vi "MT Demodulate MSK.vi"(0 "input complex waveform":T1={"t0"=0.0, "dt"=1.0, "Y"=[]} {"Y" format="%.3f"; "dt" format="%^.2e"; "t0" format="%.4f"}, 5 "MSK system parameters":T4={"differential encoding enable"=enum."enable", "samples per symbol (16)"=16}, 7 "matched filter coefficients":dbl[](array[numeric]) format="%.2f", 9 "synchronization parameters":T3 {"sync sequence" format="%.2f"}, 11 "error in (no error)":errorcluster, 12 "pulse shaping filter coefficients":dbl[](array[numeric]) format="%.2f", 13 "reset? (T)":bool=TRUE) -> (3 "detected complex waveform":cluster{"t0":dbl, "dt":dbl, "Y":cdb[]} {"Y" format="%.3f"; "dt" format="%^.2e"; "t0" format="%.4f"}, 4 "recovered complex waveform":T1 {"Y" format="%.3f"; "dt" format="%^.2e"; "t0" format="%.4f"}, 6 "output bit stream":i8[](array[numeric]), 8 "measurements":T2 {"frequency drift (Hz)" format="%.2f"; "frequency offset (Hz)" format="%.2f"}, 10 "sync found index (symbols)":dbl format="%.4f", 15 "error out":errorcluster)   [LabVIEW 2020, in "niDMT.lvlib"]
doc: "Demodulates an minimum shift keying (MSK)-modulated complex baseband waveform and returns the time-aligned oversampled complex waveform, the ideal oversampled waveform, the demodulated bit stream, and the results of offset and drift measurements. This VI attempts to remove carrier and phase offset by locking to the carrier signal."
uses:
  <vilib>/addons/Modulation/niDMT.lvlib
  <vilib>/addons/Modulation/Analog/controls/Complex Data Waveform.ctl
  <vilib>/addons/Modulation/Analog/MT Resample (Complex Cluster).vi
  <vilib>/addons/Modulation/Analog/support/Validators/mod_Fractional Resample Validate.vi
  <vilib>/addons/Modulation/Analog/support/Validators/mod_Check Flush State.vi
  <vilib>/addons/Modulation/Analog/support/mod_FractionalResampler.vi
  <vilib>/addons/Modulation/Analog/support/mod_Integer Rate Interpolation.vi
  <vilib>/addons/Modulation/Analog/support/Validators/mod_Validate Complex Waveform.vi
  <vilib>/addons/Modulation/Analog/support/mod_PerformResampling.vi
  <vilib>/addons/Modulation/Analog/support/Validators/mod_WFErrorHandler.vi
  <vilib>/addons/Modulation/Digital/Support/Common/mod_Truncate FIR Filter (real).vi
  <vilib>/Utility/error.llb/Error Cluster From Error Code.vi
  <vilib>/addons/Modulation/Analog/support/mod_Resampling Factors.vi
  <vilib>/addons/Modulation/Analog/support/mod_ResamplingFilter.vi
  <vilib>/addons/Modulation/Analog/support/mod_Generate Integer Interpolation Filter.vi
  <vilib>/addons/Modulation/niAMT.lvlib
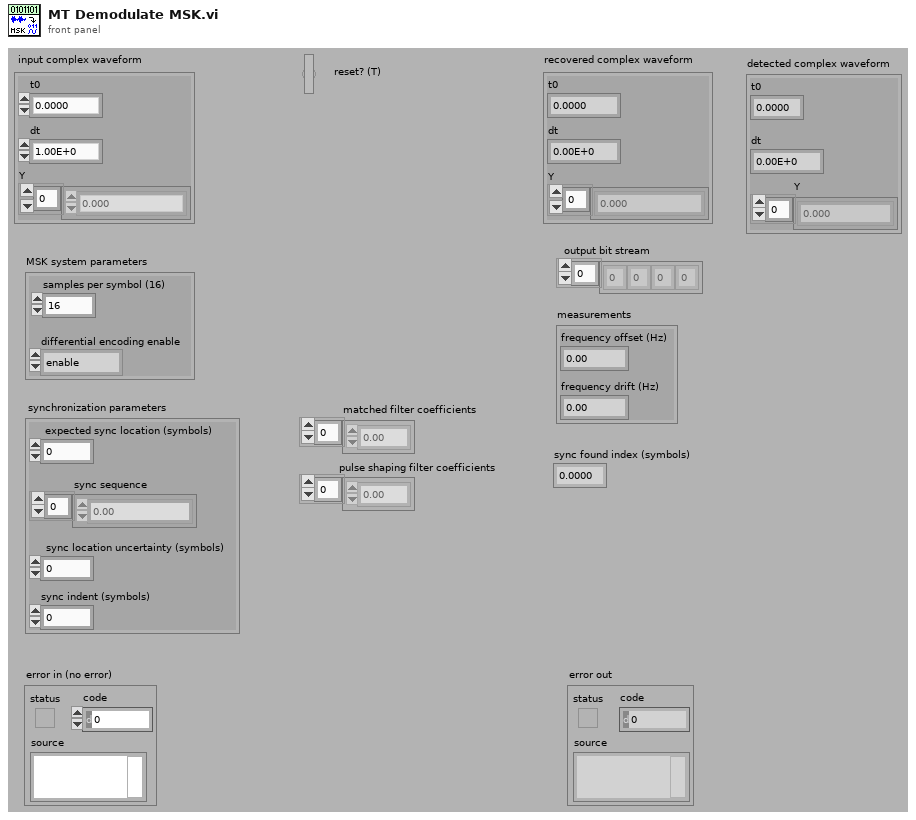
[diagram p1: front panel]
types:
  T1 = typedef "niAMT.lvlib/Complex Data Waveform.ctl" = cluster{"t0":dbl, "dt":dbl, "Y":cdb[]}
  T2 = cluster{"frequency offset (Hz)":dbl, "frequency drift (Hz)":dbl}
  T3 = cluster{"expected sync location (symbols)":i32, "sync sequence":cdb[], "sync location uncertainty (symbols)":i32, "sync indent (symbols)":i32}
  T4 = cluster{"differential encoding enable":enum16{"disable", "enable"}, "samples per symbol (16)":i32}
  T5 = enum16{"FSK", "PSK", "QAM", "MSK", "PAM", "ASK", "CPM"}
  T6 = cluster{"Frequency Estimate, Hz":dbl, "Frequency Drift, Hz":dbl}
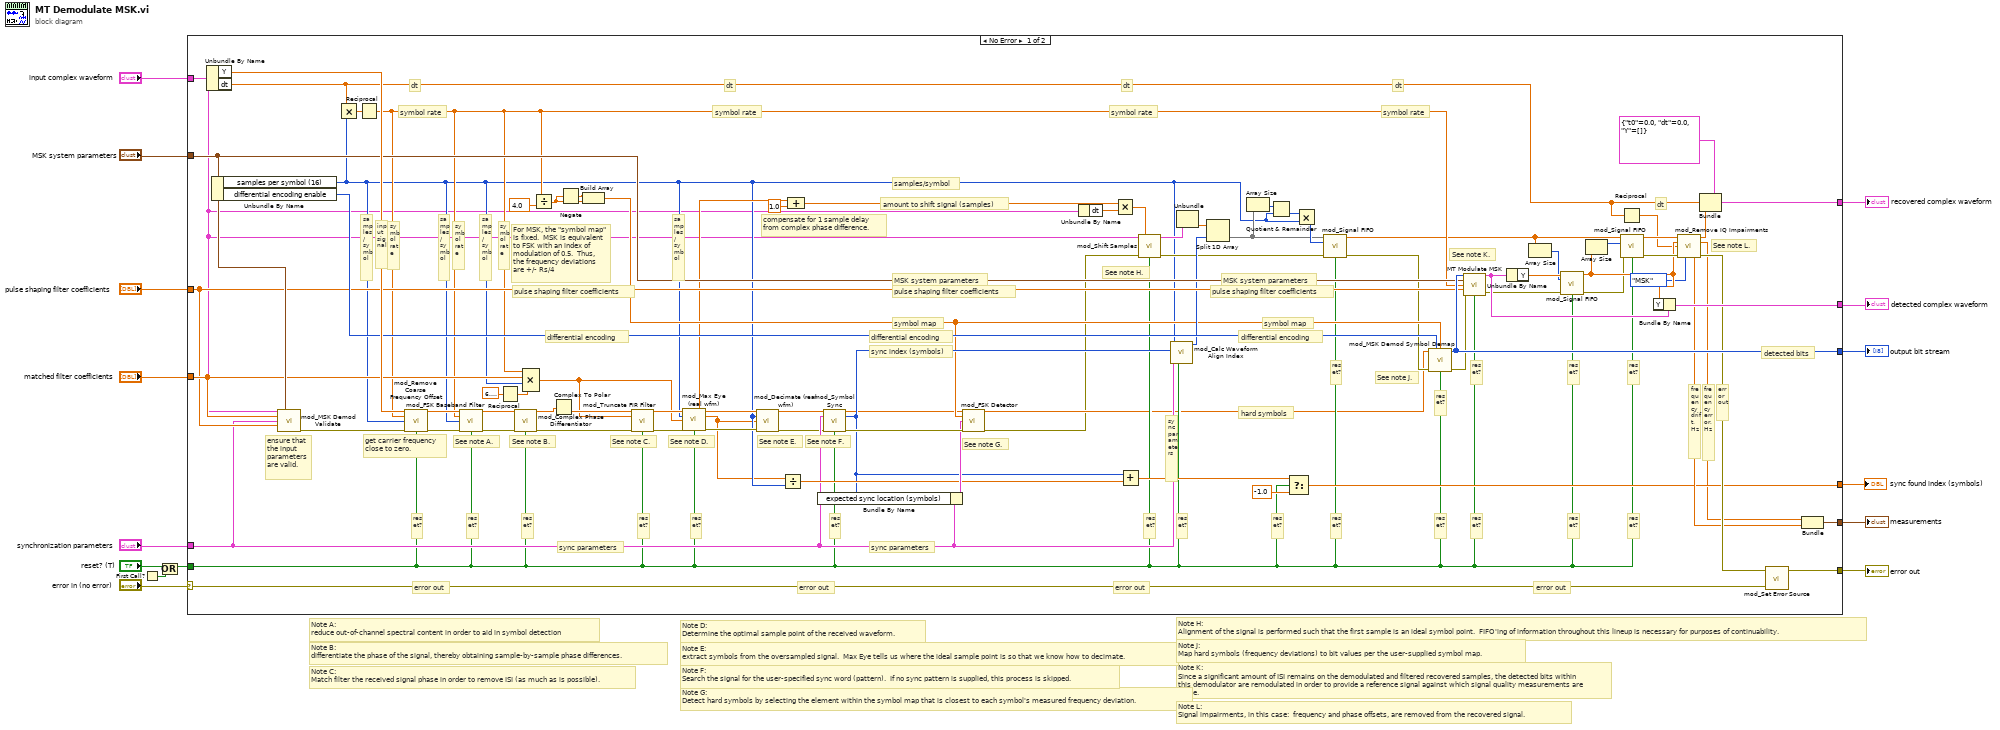
[diagram p0: block diagram]
diagram:
  # "Note A:\nreduce out-of-channel spectral content in order to aid in symbol detection"
  # "Note B:\ndifferentiate the phase of the signal, thereby obtaining sample-by-sample phase differences."
  # "Note C:\nMatch filter the received signal phase in order to remove ISI (as much as is possible)."
  # "Note D:\nDetermine the optimal sample point of the received waveform."
  # "Note E:\nextract symbols from the oversampled signal.  Max Eye tells us where the ideal sample point is so that we know how to decimate."
  # "Note F:\nSearch the signal for the user-specified sync word (pattern).  If no sync pattern is supplied, this process is skipped."
  # "Note G:\nDetect hard symbols by selecting the element within the symbol map that is closest to each symbol's measured frequency deviation."
  # "Note H:\nAlignment of the signal is performed such that the first sample is an ideal symbol point.  FIFO'ing of information throughout this lineup is necessary for purposes of continuability."
  # "Note J:\nMap hard symbols (frequency deviations) to bit values per the user-supplied symbol map."
  # "Note K:\nSince a significant amount of ISI remains on the demodulated and filtered recovered samples, the detected bits within this demodulator are remodulated in order to provide a reference signal against which signal quality measurements are made."
  # "Note L:\nSignal impairments, in this case:  frequency and phase offsets, are removed from the recovered signal."
  n1 = First Call?() -> (First Call?: T/F=w3:bool)
  n2 = Or(x="reset? (T)", y=w3) -> (x .or. y?=w1:bool)
  n3 = case shown="No Error" "error in (no error)" {
    selector: "error in (no error)" -> [w80 w98]
    tunnel: [w81 w98] -> w7
    tunnel: "synchronization parameters" -> [w63 _]
    tunnel: "matched filter coefficients" -> [w67 _]
    tunnel: "MSK system parameters" -> [w68 _]
    tunnel: "pulse shaping filter coefficients" -> [w66 _]
    tunnel: [w37 _] -> w8
    tunnel: "input complex waveform" -> [w17 _]
    tunnel: [w91 _] -> w9
    tunnel: [w88 _] -> w6
    tunnel: w1 -> [w31 _]
    tunnel: [w76 _] -> w5
    tunnel: [w72 _] -> w4
    frame No Error {
      # "sync parameters"
      # "sync parameters"
      # "sync parameters"
      # "error out"
      # "error out"
      # "error out"
      # "error out"
      # "error out"
      # "frequency error, Hz"
      # "frequency drift, Hz"
      # "samples/symbol"
      # "samples/symbol"
      # "reset?"
      # "reset?"
      # "reset?"
      # "reset?"
      # "reset?"
      # "reset?"
      # "reset?"
      # "reset?"
      # "reset?"
      # "reset?"
      # "reset?"
      # "reset?"
      # "reset?"
      # "reset?"
      # "reset?"
      # "reset?"
      # "reset?"
      # "reset?"
      # "reset?"
      # "detected bits"
      # "hard symbols"
      # "MSK system parameters"
      # "pulse shaping filter coefficients"
      # "symbol map"
      # "differential encoding"
      # "pulse shaping filter coefficients"
      # "differential encoding"
      # "input signal"
      # "symbol rate"
      # "symbol rate"
      # "samples/symbol"
      # "samples/symbol"
      # "symbol rate"
      # "sync index (symbols)"
      # "amount to shift signal (samples)"
      # "samples/symbol"
      # "differential encoding"
      # "dt"
      # "symbol rate"
      # "dt"
      # "dt"
      # "symbol rate"
      # "MSK system parameters"
      # "pulse shaping filter coefficients"
      # "symbol map"
      # "symbol rate"
      # "dt"
      # "dt"
      # "For MSK, the \"symbol map\" is fixed.  MSK is equivalent to FSK with an index of modulation of 0.5.  Thus, the frequency deviations are +/- Rs/4"
      # "compensate for 1 sample delay\nfrom complex phase difference."
      # "See note A."
      # "See note B."
      # "ensure that\nthe input\nparameters\nare valid."
      # "get carrier frequency\nclose to zero."
      # "See note D."
      # "See note E."
      # "See note C."
      # "See note F."
      # "See note G."
      # "See note H."
      # "See note J."
      # "See note K."
      # "See note L."
      # "symbol rate"
      n4 = Unbundle By Name(w17) -> ("Y"=w87:cdb[], "dt"=w24:dbl)
      n5 = Unbundle By Name(w68) -> ("samples per symbol (16)"=w29:i32, "differential encoding enable"=w71:enum16{"disable", "enable"})
      n6 = call <vilib>:"mod_MSK Demod Validate.vi"("Input Complex Waveform"=w17, "MSK System Parameters"=w68, "Matched Filter Coefficients"=w67, "Synchronization Parameters"=w63, "Pulse Shaping Filter Coefficients"=w66) -> ("error out"=w69:errorcluster)  [unwired: 10 out]
      n7 = Multiply(x=w24, y=w29) -> (x*y=w89:dbl)
      n8 = Reciprocal(x=w89) -> (1/x=w30:dbl)
      n9 = call <vilib>:"mod_Remove Coarse Frequency Offset.vi"("Signal In"=w87, "Symbol Rate, Hz"=w30, "Samples Per Symbol (16)"=w29, "error in (no error)"=w69, "Reset? (T)"=w31) -> ("Signal Out"=w33:cdb[], "error out"=w35:errorcluster)  [unwired: 9 out]
      n10 = call <vilib>:"mod_FSK Baseband Filter.vi"("Signal In"=w33, "Symbol Rate, Hz"=w30, "Samples Per Symbol (16)"=w29, "error in (no error)"=w35, "Reset? (T)"=w31) -> ("Signal Out"=w32:cdb[], "error out"=w34:errorcluster)  [unwired: 9 in]
      n11 = Reciprocal(x=6.283185307179586) -> (1/x=w86:dbl)
      n12 = call <vilib>:"mod_Complex Phase Differentiator.vi"("Signal In"=w32, "error in (no error)"=w34, "Reset? (T)"=w31) -> ("Signal Out"=w54:cdb[], "error out"=w96:errorcluster)  [unwired: 11 in]
      n13 = Compound Arithmetic op=MULTIPLY(w30, w67, w29, w86) -> (w41:dbl[])
      n14 = Divide(x=w30, y=4.0) -> (x/y=w74:dbl)
      n15 = Complex To Polar(r * e^(i*theta)=w54) -> (theta=w90:dbl[])  [unwired: 1 out]
      n16 = Negate(x=w74) -> (-x=w73:dbl)
      n17 = Build Array(w73, w74) -> (w43:dbl[])
      n18 = call-poly <vilib>:"mod_Truncate FIR Filter.vi"("Signal In"=w90, "Filter Coefficients"=w41, "error in (no error)"=w96, "Reset? (T)"=w31) -> ("Signal Out"=w92:dbl[], "error out"=w95:errorcluster)  [unwired: 8 in, 2 out]
      n19 = call <vilib>:"mod_Max Eye (real wfm).vi"("Signal In"=w92, "Samples Per Symbol (16)"=w29, "Filter Coefficients"=w41, "error in (no error)"=w95, "Reset? (T)"=w31) -> ("Waveform Alignment Offset"=w42:dbl, "Signal Out"=w48:dbl[], "Optimal Offset (samples)"=w19:dbl, "error out"=w94:errorcluster)  [unwired: 6 in, 1 out]
      n20 = call <vilib>:"mod_Decimate (real wfm).vi"("Signal In"=w48, "Samples Per Symbol (16)"=w29, "Offset"=w19, "error in (no error)"=w94) -> ("Signal Out"=w44:dbl[], "error out"=w28:errorcluster)  [unwired: 10 in]
      n21 = Divide(x=w19, y=w29) -> (x/y=w65:dbl)
      n22 = Compound Arithmetic op=ADD(w42, 1.0 ("value")) -> (w40:dbl)
      n23 = call <vilib>:"mod_Symbol Sync.vi"("Signal In"=w44, "Synchronization Parameters"=w63, "error in (no error)"=w28, "Reset? (T)"=w31) -> ("Signal Out"=w36:cdb[], "Sync Location (symbols)"=w61:i32, "error out"=w97:errorcluster)  [unwired: 9 out]
      n24 = Bundle By Name(cluster=w63, "expected sync location (symbols)"=w61) -> (w83:T3)
      n25 = call <vilib>:"mod_FSK Detector.vi"("Symbols"=w36, "Symbol Map"=w43, "Synchronization Parameters"=w83, "error in (no error)"=w97) -> ("Detected Symbols"=w22:dbl[], "error out"=w18:errorcluster)  [unwired: 1 in, 9 out]
      n26 = Unbundle By Name(w17) -> ("dt"=w16:dbl)
      n27 = Multiply(x=w40, y=w16) -> (x*y=w79:dbl)
      n28 = Add(x=w61, y=w65) -> (x+y=w39:dbl)
      n29 = call <vilib>:"mod_Shift Samples.vi"("Input Complex Waveform"=w17, "Initial Sample Offset, sec"=w79, "error in (no error)"=w18, "Reset? (T)"=w31) -> ("Output Complex Waveform"=w84:T1, "error out"=w56:errorcluster)  [unwired: 10 in]
      n30 = call <vilib>:"mod_Calc Waveform Align Index.vi"("Reset? (T)"=w31, "Synchronization Parameters"=w63, "Sync Location, symbols"=w61, "Samples Per Symbol (16)"=w29) -> ("align index, samples"=w62:i32)  [unwired: 7 out]
      n31 = Unbundle(w84) -> ("Y"=w85:cdb[])  [unwired: 2 out]
      n32 = Split 1D Array(array=w85, index=w62) -> (second subarray=w57:cdb[])  [unwired: 1 out]
      n33 = Array Size(array=w57) -> (size(s)=w60:i32)
      n34 = Quotient & Remainder(x=w60, y=w29) -> (floor(x/y)=w59:i32)  [unwired: 1 out]
      n35 = Select(t=w39, s=w31, f=-1.0) -> (s? t:f=w37:dbl)
      n36 = Multiply(x=w59, y=w29) -> (x*y=w58:i32)
      n37 = call <vilib>:"mod_Signal FIFO.vi"("Signal In"=w57, "Output Length"=w58, "error in (no error)"=w56, "Reset? (T)"=w31) -> ("Signal Out"=w26:cdb[], "error out"=w27:errorcluster)  [unwired: 10 out]
      n38 = call <vilib>:"mod_MSK Demod Symbol Demap.vi"("Symbols In"=w22, "Differential Encoding Enable"=w71, "Symbol Map"=w43, "error in (no error)"=w27, "Reset? (T)"=w31) -> ("Bits Out"=w91:i8[], "error out"=w47:errorcluster)  [unwired: 9 out]
      n39 = call <vilib>:"MT Modulate MSK.vi"("input bit stream"=w91, "MSK system parameters"=w68, "symbol rate (Hz)"=w30, "pulse shaping filter coefficients"=w66, "error in (no error)"=w47, "reset? (T)"=w31) -> ("output complex waveform"=w77:T1, "error out"=w46:errorcluster)  [unwired: 1 in, 7 out]
      n40 = Unbundle By Name(w77) -> ("Y"=w78:cdb[])
      n41 = Array Size(array=w26) -> (size(s)=w55:i32)
      n42 = call <vilib>:"mod_Signal FIFO.vi"("Signal In"=w78, "Output Length"=w55, "error in (no error)"=w46, "Reset? (T)"=w31) -> ("Signal Out"=w49:cdb[], "error out"=w45:errorcluster)  [unwired: 10 out]
      n43 = Array Size(array=w49) -> (size(s)=w51:i32)
      n44 = Reciprocal(x=w24) -> (1/x=w23:dbl)
      n45 = call <vilib>:"mod_Signal FIFO.vi"("Signal In"=w26, "Output Length"=w51, "error in (no error)"=w45, "Reset? (T)"=w31) -> ("Signal Out"=w53:cdb[], "error out"=w52:errorcluster)  [unwired: 10 out]
      n46 = Bundle By Name(cluster=w77, "Y"=w49) -> (w72:T1)
      n47 = call <vilib>:"mod_Remove IQ Impairments.vi"("Received Signal In"=w53, "Reference Signal"=w49, "Signal Rate, Hz"=w23, "error in (no error)"=w52, "Modulation Type"=T5."MSK") -> ("Received Signal Out"=w50:cdb[], "Frequency Estimate, Hz"=w25:dbl, "Frequency Drift, Hz"=w64:dbl, "error out"=w70:errorcluster)  [unwired: 1 in, 6 out]
      n48 = Bundle(cluster=T1 {"t0"=0.0, "dt"=0.0, "Y"=[]} ("Recovered Complex Waveform"), "dt"=w24, "Y"=w50) -> (w76:T1)  [unwired: 1 out]
      n49 = call <vilib>:"mod_Set Error Source.vi"("initial error in (no error)"=w80, "final error in (no error)"=w70) -> ("error out"=w81:errorcluster)  [unwired: 3 out]
      n50 = Bundle("Frequency Estimate, Hz"=w25, "Frequency Drift, Hz"=w64) -> (w88:T6)  [unwired: 1 out]
    }
    frame Error {
    }
  }
  "error out" <- w7
  "sync found index (symbols)" <- w8
  "output bit stream" <- w9
  "measurements" <- w6
  "recovered complex waveform" <- w5
  "detected complex waveform" <- w4
